vi "FindDataFrom2DArray.vi"(9 "column index":u16, 10 "search string":string, 11 "array in":string[][](array[string])) -> (2 "is empty?":bool, 3 "array out":string[][](array[string]))   [LabVIEW 2018, in "Library-Ctrl.lvlib"]
uses:
  Library-Ctrl.lvlib
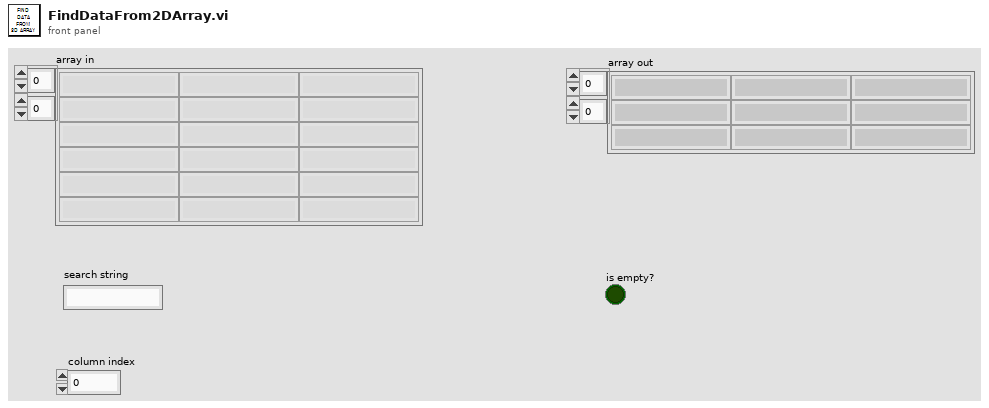
[diagram p1: front panel]
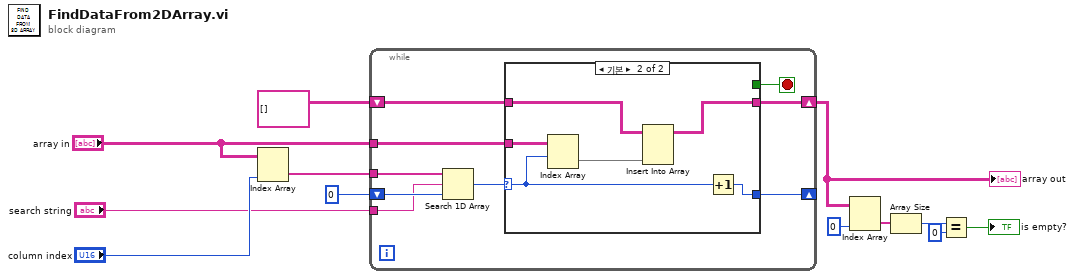
[diagram p0: block diagram]
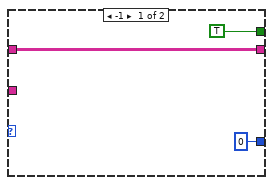
[diagram p2: hidden frame]
diagram:
  n1 = Index Array(array="array in", index (col)="column index") -> (element=w11:string[])  [unwired: 1 in]
  n2 = while {
    tunnel: w11 -> [w17]
    shift-right: [w15] -> _
    shift-left: 0 ("시작 인덱스(0)") -> [w21]
    tunnel: "search string" -> [w20]
    shift-right: [w16] -> w7
    shift-left: string[][] [] ("result") -> [w18]
    tunnel: "array in" -> [w13]
    stop <- w14 stop-if-true
    n3 = Search 1D Array(1D array=w17, element=w20, start index (0)=w21) -> (index of element=w19:i32)
    n4 = case shown="기본" w19 {
      selector: w19 -> [_ w26]
      tunnel: w18 -> [w24 w30]
      tunnel: [w24 w29] -> w16
      tunnel: [0 w28] -> w15
      tunnel: [TRUE _] -> w14
      tunnel: w13 -> [_ w27]
      frame -1 {
      }
      frame Default {
        n5 = Index Array(array=w27, index (row)=w26) -> (element=w25:string[])  [unwired: 1 in]
        n6 = Insert Into Array(array=w30, new element=w25) -> (w29:string[][])  [unwired: 2 in]
        n7 = Increment(x=w26) -> (x+1=w28:i32)
      }
    }
  }
  "array out" <- w7
  n8 = Index Array(array=w7, index (col)=0 ("비활성화된 인덱스 (열)")) -> (element=w5:string[])  [unwired: 1 in]
  n9 = Array Size(array=w5) -> (size(s)=w4:i32)
  n10 = Equal?(x=w4, y=0) -> (x = y?=→"is empty?":bool)
